vi "Build_Asylum_GetGroupRanges.vi"(8 "error in (no error)":errorcluster, 10 "textWave":string, 11 "groupName":string) -> (0 "error out":errorcluster, 3 "Command":string)   [LabVIEW 2019]
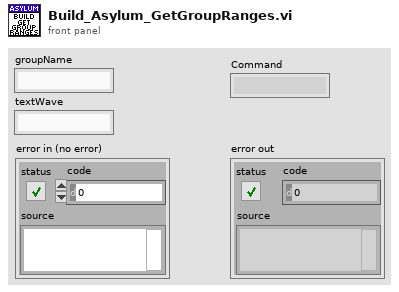
[diagram p1: front panel]
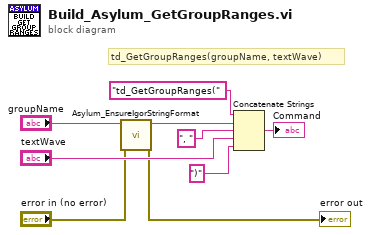
[diagram p0: block diagram]
diagram:
  # "td_GetGroupRanges(groupName, textWave)"
  n1 = call "Asylum_EnsureIgorStringFormat.vi"("error in (no error)"="error in (no error)", "Value"="groupName") -> ("error out"=→"error out":errorcluster, "Value"=w3:string)  [unwired: 8 in]
  n2 = Concatenate Strings("td_GetGroupRanges(", w3, ", " ("string"), "textWave", ")" ("string")) -> (→"Command":string)
